vi "ControlwordToCommand.vi"(11 "Data_In":u16 format="%.0b") -> (3 "Device Control Command":T1)   [LabVIEW 2017, in "WordManipulationLibrary.lvlib"]
uses:
  WordManipulationLibrary.lvlib
  Controlword_Commands.ctl
  Bit Manipulation.lvlib
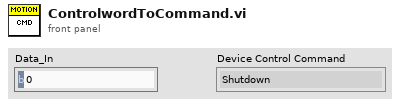
[diagram p1: front panel]
types:
  T1 = typedef "WordManipulationLibrary.lvlib/Controlword_Commands.ctl" = enum16{"Shutdown", "Switch On", "Disable Voltage", "Quick Stop", "Disable Op", "Enable Op", "Fault Reset", "Error"}
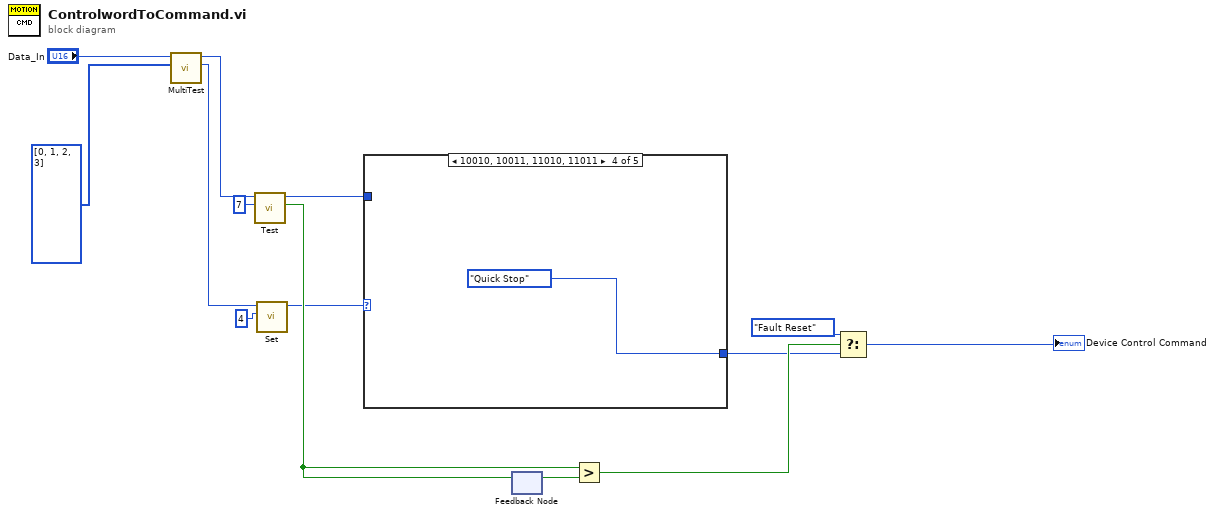
[diagram p0: block diagram]
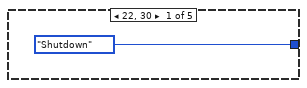
[diagram p2: hidden frame]
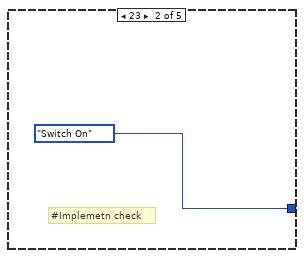
[diagram p3: hidden frame]
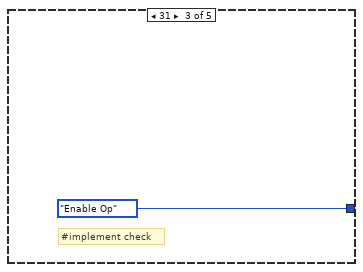
[diagram p4: hidden frame]
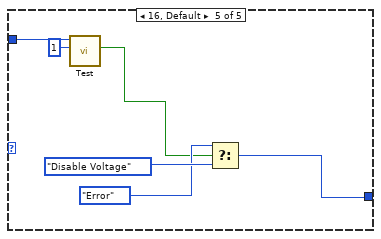
[diagram p5: hidden frame]
diagram:
  n1 = call "MultiTest.vi"("Array"=u8[] [0, 1, 2, 3], "Data_In"="Data_In") -> ("MaskedWord"=w3:u32, "Data_Out"=w2:u16)  [unwired: 8 in]
  n2 = call "Test.vi"("Bit to test"=u8 7, "Data_In"=w2) -> ("bit value"=w12:bool, "Data_Out"=w14:u16)  [unwired: 8 in]
  n3 = call "Set.vi"("Bit to set"=u8 4, "Data_In"=w3) -> ("Data_Out"=w11:u16)  [unwired: 9 in]
  n4 = case shown="10010, 10011, 11010, 11011" w11 {
    tunnel: [Controlword_Commands."Shutdown" ("Device Control Command") Controlword_Commands."Switch On" ("Device Control Command") Controlword_Commands."Enable Op" ("Device Control Command") Controlword_Commands."Quick Stop" ("Device Control Command") w24] -> w6
    tunnel: w14 -> [_ _ _ _ w21]
    frame 22, 30 {
    }
    frame 23 {
      # "#Implemetn check"
    }
    frame 31 {
      # "#implement check"
    }
    frame 18, 19, 26, 27 {
    }
    frame 16, Default {
      n5 = call "Test.vi"("Bit to test"=u8 1, "Data_In"=w21) -> ("bit value"=w19:bool)  [unwired: 8 in, 1 out]
      n6 = Select(t=Controlword_Commands."Error", s=w19, f=Controlword_Commands."Disable Voltage" ("Device Control Command")) -> (s? t:f=w24:T1)
    }
  }
  n7 = feedback #1() -> (w8:bool)  [unwired: 1 in]
  n8 = feedback-in #1(w12) -> ()
  n9 = Greater?(x=w12, y=w8) -> (0:w9:bool)
  n10 = Select(t=Controlword_Commands."Fault Reset" ("Device Control Command"), s=w9, f=w6) -> (s? t:f=→"Device Control Command":T1)
